vi "Filter FPGA by Tag.vi"(8 "error in (no error)":errorcluster, 10 "FPGA Personality Tag":string, 11 "FPGA Personality File Paths":path[](array[path])) -> (0 "error out":errorcluster, 2 "First Path":path, 3 "Filtered FPGA Personality File Paths":path[](array[path]))   [LabVIEW 2021, in "Personality.lvlib"]
doc: "Filters the FPGA personality paths with specified FPGA personality tag."
uses:
  <vilib>/myRIO/Common/FPGA Personality Framework/Personality.lvlib
  <vilib>/xml/Load XML File.vi
  <vilib>/xml/Close Reference(Node).vi
  <vilib>/xml/NI_XML.lvlib
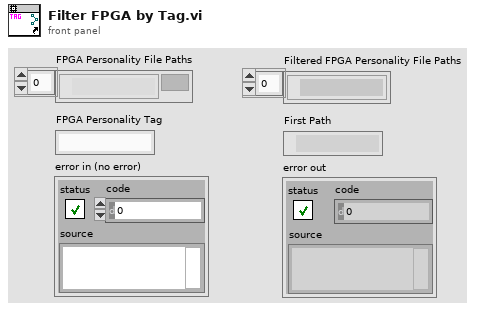
[diagram p1: front panel]
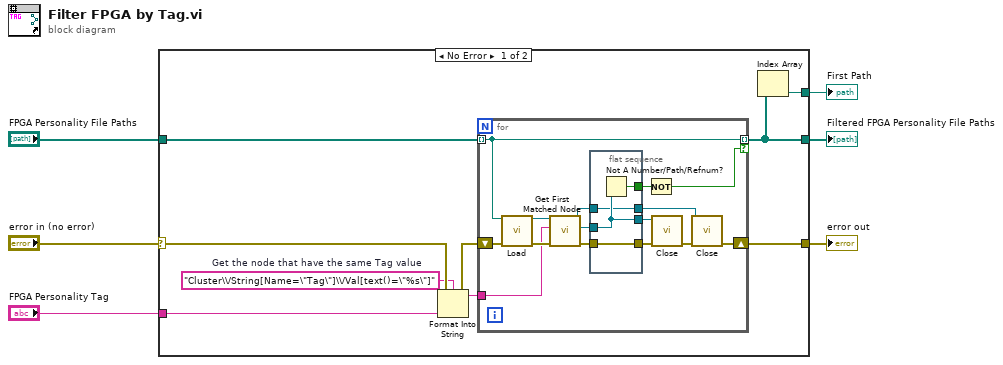
[diagram p0: block diagram]
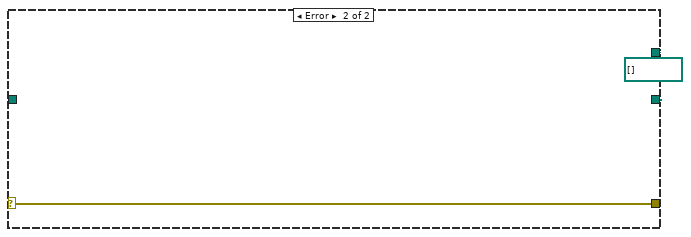
[diagram p2: hidden frame]
diagram:
  n1 = case shown="No Error" "error in (no error)" {
    selector: "error in (no error)" -> [w15 w37]
    tunnel: "FPGA Personality File Paths" -> [w8 _]
    tunnel: [w9 w37] -> w5
    tunnel: "FPGA Personality Tag" -> [w14 _]
    tunnel: [w7 path[] []] -> w2
    tunnel: [w12 path "" ("FPGA Personality File Path")] -> w1
    frame No Error {
      w13 = "Cluster\\/String[Name=\"Tag\"]\\/Val[text()=\"%s\"]"  # Get the node that have the same Tag value
      n2 = Format Into String(format string=w13, error in=w15, w14) -> (resulting string=w10:string, error out=w11:errorcluster)  [unwired: 1 in]
      n3 = for {
        shift-right: [w23] -> w9
        shift-left: w11 -> [w29]
        tunnel: w8 -> [w25] mode=indexing
        tunnel: w10 -> [w26]
        tunnel: [w25] -> w7 mode=indexing if=w24
        n4 = call-poly <vilib>:"Load.vi"("path to XML document"=w25, "error in (no error)"=w29) -> ("DOM document out"=w30:refnum<k20>, "error out"=w28:errorcluster)  [unwired: 11 in, 1 out]
        n5 = call <vilib>:"Get First Matched Node.vi"("error in (no error)"=w28, "XPath expression"=w26, "node in"=w30) -> ("error out"=w22:errorcluster, "node result"=w21:refnum<k20>, "node out"=w17:refnum<k20>)  [unwired: 6 in]
        n6 = flat-sequence {
          tunnel: [w34] -> w18
          tunnel: w22 -> [w32]
          tunnel: w21 -> [w33]
          tunnel: [w33] -> w20
          tunnel: [w32] -> w19
          tunnel: w17 -> [w31]
          tunnel: [w31] -> w16
          frame #0 {
            n7 = Not A Number/Path/Refnum?(number/path/refnum=w33) -> (NaN/Path/Refnum?=w34:bool)
          }
        }
        n8 = Not(x=w18) -> (.not. x?=w24:bool)
        n9 = call-poly <vilib>:"Close.vi"("error in (no error)"=w19, "node"=w20) -> ("error out"=w27:errorcluster)  [unwired: 7 in]
        n10 = call-poly <vilib>:"Close.vi"("error in (no error)"=w27, "node"=w16) -> ("error out"=w23:errorcluster)  [unwired: 7 in]
      }
      n11 = Index Array(array=w7) -> (element=w12:path)  [unwired: 1 in]
    }
    frame Error {
    }
  }
  "First Path" <- w1
  "Filtered FPGA Personality File Paths" <- w2
  "error out" <- w5
